vi "Apply Column Setup After Binding.vi"(7 "DataTable":refnum<class "DataTable.lvclass">, 8 "error in (no error)":errorcluster, 11 "DataGridView in":refnum<class "DataGridView.lvclass">) -> (0 "error out":errorcluster, 3 "DataGridView out":refnum<class "DataGridView.lvclass">)   [LabVIEW 2016, in "DataGrid.lvlib" / "DataGridView.lvclass"]
doc: "This is called after populating the datagridview (via binding its DataTable) so that the custom datatypes can be setup for the columns that require it. This is only needed if you are using <B>Buttons</B> or <B>Combos</B> as all other types are completely automatic."
uses:
  <userlib>/LabVIEWdotNetDataGrid/source/DataGridView/DataGridView.lvclass
  <userlib>/LabVIEWdotNetDataGrid/source/DataTable/DataTable.lvclass
  <userlib>/LabVIEWdotNetDataGrid/source/DataGridView/DataGridView.lvclass/DataGridView.ctl
  System.Windows.Forms
  <userlib>/LabVIEWdotNetDataGrid/source/GridColumn/GridColumn.lvclass/GridColumn.ctl
  <userlib>/LabVIEWdotNetDataGrid/source/GridColumn/Read Params.vi
  <userlib>/LabVIEWdotNetDataGrid/source/GridColumn/Read Caption.vi
  <userlib>/LabVIEWdotNetDataGrid/source/GridColumn/Read Name.vi
  <userlib>/LabVIEWdotNetDataGrid/source/GridColumn/Read AutoSizeMode.vi
  <userlib>/LabVIEWdotNetDataGrid/source/GridColumn/Read FillWeight.vi
  <userlib>/LabVIEWdotNetDataGrid/source/GridColumn/Read datatype.vi
  <userlib>/LabVIEWdotNetDataGrid/source/GridColumn/Read Tooltip.vi
  <userlib>/LabVIEWdotNetDataGrid/source/GridColumn/Read ReadOnly.vi
  <userlib>/LabVIEWdotNetDataGrid/source/GridColumn/Read Visible.vi
  <userlib>/LabVIEWdotNetDataGrid/source/GridColumn/GridColumn.lvclass
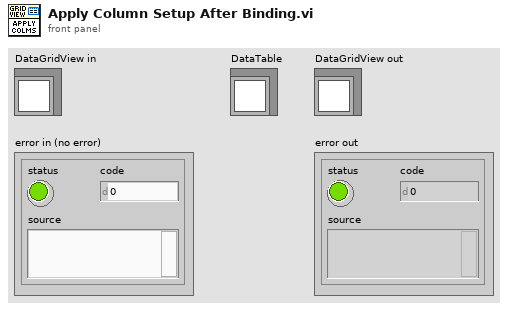
[diagram p1: front panel]
types:
  T1 = typedef "DataGrid.lvlib/GridColumn.lvclass/ColumnType.ctl" = enum16{"string", "image", "check", "numeric", "timestamp", "button", "combo", "link"}
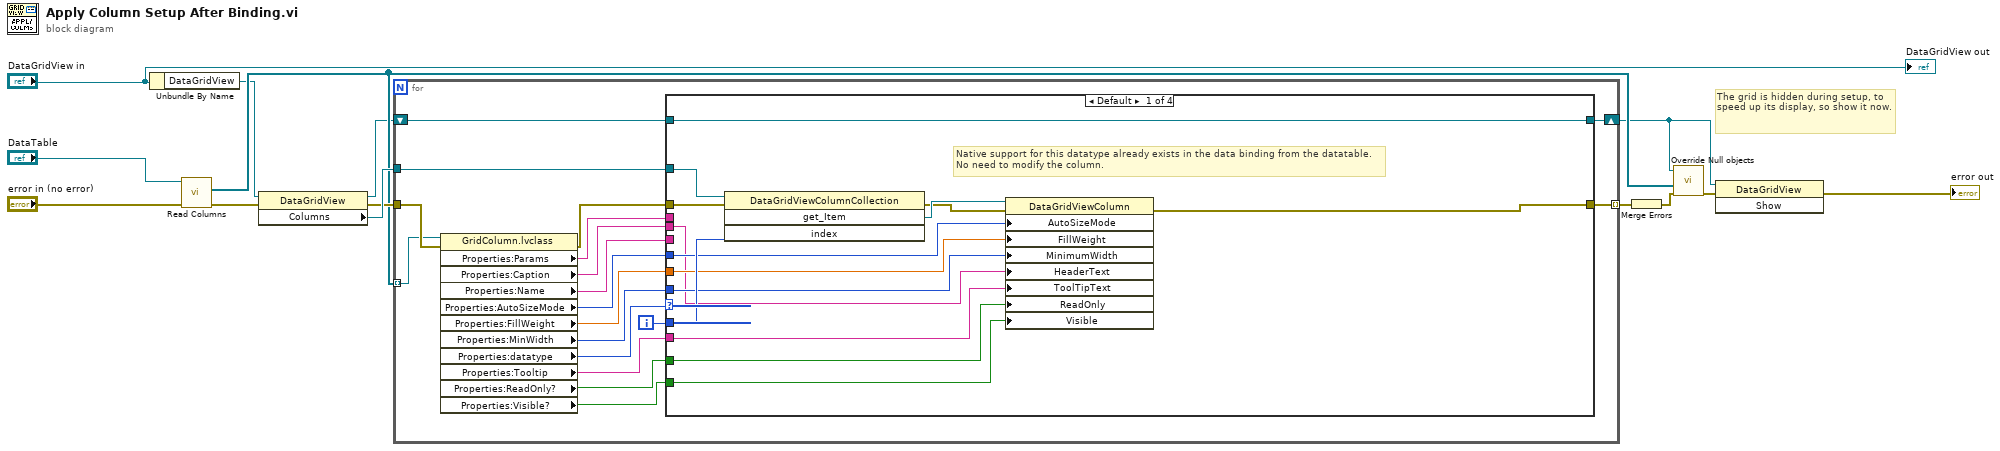
[diagram p0: block diagram]
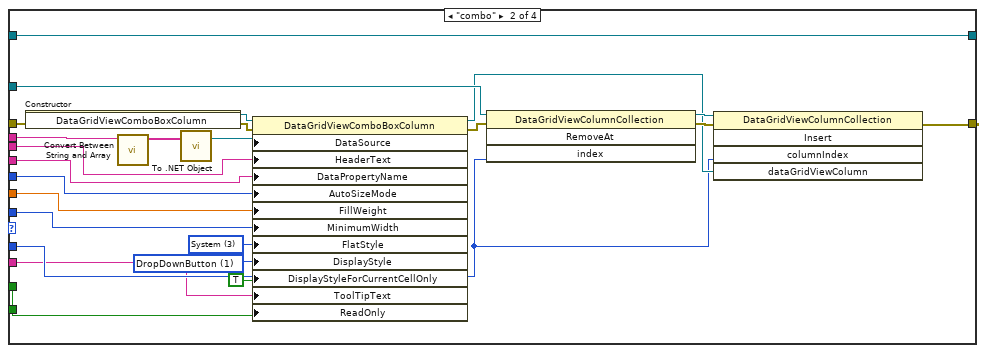
[diagram p2: hidden frame]
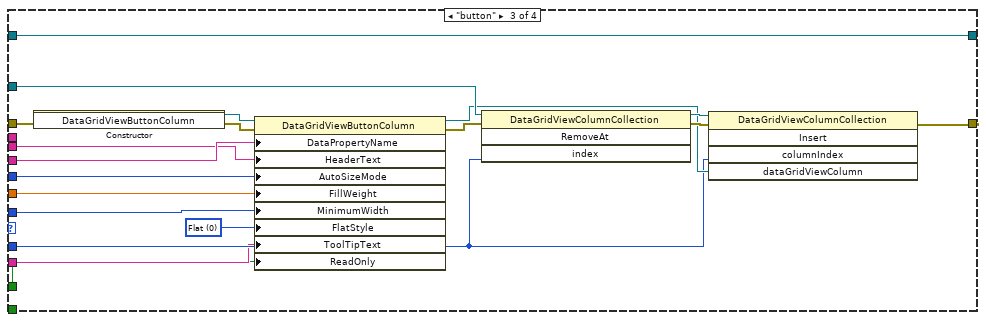
[diagram p3: hidden frame]
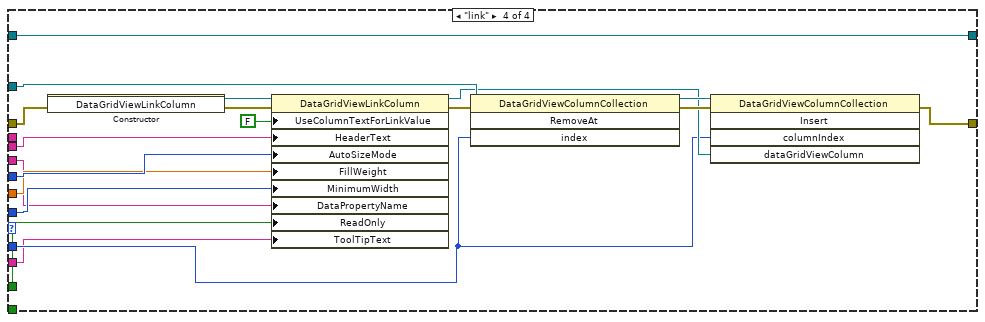
[diagram p4: hidden frame]
diagram:
  # "The grid is hidden during setup, to speed up its display, so show it now."
  n1 = Unbundle By Name("DataGridView in") -> ("DataGridView"=w1:refnum<k24>)
  n2 = call <userlib>:"Read Columns.vi"("error in (no error)"="error in (no error)", "DataTable in"="DataTable") -> ("error out"=w7:errorcluster, "Columns"=w6:refnum<class "GridColumn.lvclass">[])  [unwired: 7 in, 1 out]
  n3 = property class="DataGridView"(reference=w1, error in=w7) -> (reference out=w3:refnum<k24>, error out=w10:errorcluster, "Columns"=w12:refnum<k24>)
  n4 = for {
    tunnel: w12 -> [w32]
    tunnel: [w31] -> w13 mode=indexing
    tunnel: w10 -> [w22]
    tunnel: w6 -> [w21] mode=indexing
    shift-right: [w18] -> w2
    shift-left: w3 -> [w19]
    i -> [w30]
    n5 = property class="GridColumn.lvclass"(reference=w21, error in=w22) -> (error out=w23:errorcluster, "Properties:Params"=w29:string, "Properties:Caption"=w20:string, "Properties:Name"=w28:string, "Properties:AutoSizeMode"=w27:i32, "Properties:FillWeight"=w24:sgl, "Properties:MinWidth"=w26:i32, "Properties:datatype"=w25:T1, "Properties:Tooltip"=w17:string, "Properties:ReadOnly?"=w16:bool, "Properties:Visible?"=w15:bool)  [unwired: 1 out]
    n6 = case shown="Default" w25 {
      tunnel: w32 -> [w46 w68 w87 w99]
      tunnel: [w38 w49 w73 w98] -> w31
      tunnel: w30 -> [w45 w50 w74 w92]
      tunnel: w28 -> [_ w55 w79 w95]
      tunnel: w29 -> [_ w58 _ _]
      tunnel: w26 -> [w40 w59 w83 w102]
      tunnel: w24 -> [w41 w60 w82 w103]
      tunnel: w27 -> [w42 w61 w81 w104]
      tunnel: w23 -> [w39 w57 w80 w108]
      tunnel: w20 -> [w37 w56 w78 w94]
      tunnel: w19 -> [w36 w54 w77 w93]
      tunnel: [w36 w54 w77 w93] -> w18
      tunnel: w17 -> [w35 w48 w72 w91]
      tunnel: w16 -> [w34 w47 w71 w90]
      tunnel: w15 -> [w33 _ _ _]
      frame Default {
        # "Native support for this datatype already exists in the data binding from the datatable.\nNo need to modify the column."
        n7 = invoke class="DataGridViewColumnCollection" method="get_Item"(reference=w46, error in=w39, "index"=w45) -> (error out=w43:errorcluster, "get_Item"=w44:refnum<k24>)  [unwired: 1 in, 2 out]
        n8 = property class="DataGridViewColumn"(reference=w44, error in=w43, "AutoSizeMode"=w42, "FillWeight"=w41, "MinimumWidth"=w40, "HeaderText"=w37, "ToolTipText"=w35, "ReadOnly"=w34, "Visible"=w33) -> (error out=w38:errorcluster)  [unwired: 1 out]
      }
      frame "combo" {
        w52 = 1 items=["ComboBox", "DropDownButton", "Nothing"] ("DisplayStyle")
        w53 = 3 items=["Flat", "Popup", "Standard", "System"] ("FlatStyle")
        n9 = constructor class="DataGridViewComboBoxColumn"(error in=w57) -> (reference out=w70:refnum<k24>, error out=w69:errorcluster)  [unwired: 2 in, 1 out]
        n10 = call <userlib>:"Convert Between String and Array.vi"("String"=w58) -> ("String Array"=w62:string[])  [unwired: 9 in, 1 out]
        n11 = call <vilib>:"To .NET Object.vi"("anything"=w62) -> (".NET object"=w64:refnum<k24>)  [unwired: 1 in, 1 out]
        n12 = property class="DataGridViewComboBoxColumn"(reference=w70, error in=w69, "DataSource"=w64, "HeaderText"=w56, "DataPropertyName"=w55, "AutoSizeMode"=w61, "FillWeight"=w60, "MinimumWidth"=w59, "FlatStyle"=w53, "DisplayStyle"=w52, "DisplayStyleForCurrentCellOnly"=TRUE, "ToolTipText"=w48, "ReadOnly"=w47) -> (reference out=w65:refnum<k24>, error out=w63:errorcluster)
        n13 = invoke class="DataGridViewColumnCollection" method="RemoveAt"(reference=w68, error in=w63, "index"=w50) -> (reference out=w66:refnum<k24>, error out=w67:errorcluster)  [unwired: 1 in, 2 out]
        n14 = invoke class="DataGridViewColumnCollection" method="Insert"(reference=w66, error in=w67, "columnIndex"=w50, "dataGridViewColumn"=w65) -> (error out=w49:errorcluster)  [unwired: 1 in, 4 out]
      }
      frame "button" {
        w76 = 0 items=["Flat", "Popup", "Standard", "System"] ("FlatStyle")
        n15 = constructor class="DataGridViewButtonColumn"(error in=w80) -> (reference out=w89:refnum<k24>, error out=w88:errorcluster)  [unwired: 2 in, 1 out]
        n16 = property class="DataGridViewButtonColumn"(reference=w89, error in=w88, "DataPropertyName"=w79, "HeaderText"=w78, "AutoSizeMode"=w81, "FillWeight"=w82, "MinimumWidth"=w83, "FlatStyle"=w76, "ToolTipText"=w72, "ReadOnly"=w71) -> (reference out=w75:refnum<k24>, error out=w84:errorcluster)
        n17 = invoke class="DataGridViewColumnCollection" method="RemoveAt"(reference=w87, error in=w84, "index"=w74) -> (reference out=w85:refnum<k24>, error out=w86:errorcluster)  [unwired: 1 in, 2 out]
        n18 = invoke class="DataGridViewColumnCollection" method="Insert"(reference=w85, error in=w86, "columnIndex"=w74, "dataGridViewColumn"=w75) -> (error out=w73:errorcluster)  [unwired: 1 in, 4 out]
      }
      frame "link" {
        n19 = constructor class="DataGridViewLinkColumn"(error in=w108) -> (reference out=w107:refnum<k24>, error out=w106:errorcluster)  [unwired: 2 in, 1 out]
        n20 = property class="DataGridViewLinkColumn"(reference=w107, error in=w106, "UseColumnTextForLinkValue"=FALSE, "HeaderText"=w94, "AutoSizeMode"=w104, "FillWeight"=w103, "MinimumWidth"=w102, "DataPropertyName"=w95, "ReadOnly"=w90, "ToolTipText"=w91) -> (reference out=w96:refnum<k24>, error out=w97:errorcluster)
        n21 = invoke class="DataGridViewColumnCollection" method="RemoveAt"(reference=w99, error in=w97, "index"=w92) -> (reference out=w100:refnum<k24>, error out=w101:errorcluster)  [unwired: 1 in, 2 out]
        n22 = invoke class="DataGridViewColumnCollection" method="Insert"(reference=w100, error in=w101, "columnIndex"=w92, "dataGridViewColumn"=w96) -> (error out=w98:errorcluster)  [unwired: 1 in, 4 out]
      }
    }
  }
  n23 = Merge Errors(w13) -> (w5:errorcluster)
  n24 = call <userlib>:"Override Null objects.vi"("error in (no error)"=w5, "Columns"=w6, ".NET Refnum in"=w2) -> ("error out"=w4:errorcluster)  [unwired: 8 in]
  n25 = invoke class="DataGridView" method="Show"(reference=w2, error in=w4) -> (error out=→"error out":errorcluster)  [unwired: 1 in, 2 out]
  "DataGridView out" <- "DataGridView in"
